vi "scp_send.vi"() -> ()   [LabVIEW 2017]
doc: "Illustrates how to send a file to a remote server via SCP."
uses:
  libssh2/libssh2_session_handshake_tcp.vi
  libssh2/libssh2_init_default.vi
  libssh2/libssh2_session_init_ex.vi
  <vilib>/Utility/tcp.llb/TCP Get Raw Net Object.vi
  libssh2/libssh2_session_handshake_socket.vi
  libssh2/libssh2_userauth_password_ex.vi
  libssh2/libssh2_channel_write_ex.vi
  libssh2/libssh2.lvlib
panel:
  out "size(s)":i32
  in  "data":string="Lorem ipsum dolor sit amet, consetetur sadipscing elitr, sed diam nonumy eirmod tempor invidunt ut labore et dolore magna aliquyam erat, sed diam voluptua. At vero eos et accusam et justo duo dolores et ea rebum. Stet clita kasd gubergren, no sea takimata sanctus est Lorem ipsum dolor sit amet. Lorem ipsum dolor sit amet, consetetur sadipscing elitr, sed diam nonumy eirmod tempor invidunt ut labore et dolore magna aliquyam erat, sed diam voluptua. At vero eos et accusam et justo duo dolores et ea rebum. Stet clita kasd gubergren, no sea takimata sanctus est Lorem ipsum dolor sit amet."
  out "error message":string
  in  "file":string="/"
  out "error out":errorcluster
  in  "password":string
  in  "username":string
  in  "hostname":string
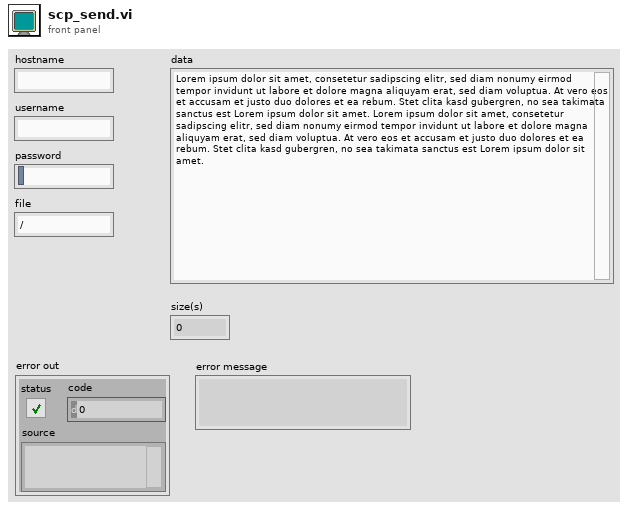
[diagram p1: front panel]
types:
  T1 = typedef "libssh2.lvlib/Session Refnum.ctl" = refnum<k1>
  T2 = typedef "libssh2.lvlib/Channel Refnum.ctl" = refnum<k1>
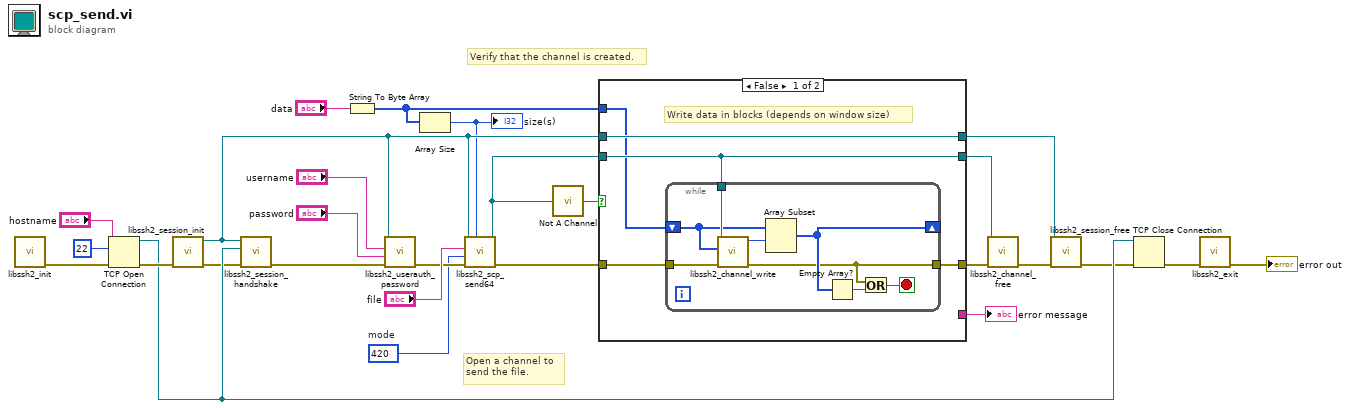
[diagram p0: block diagram]
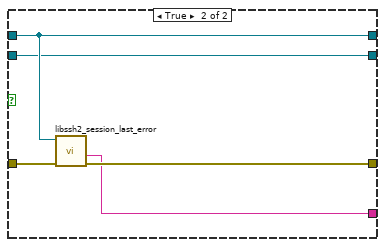
[diagram p2: hidden frame]
diagram:
  w1 = 420  # mode
  # "Verify that the channel is created."
  # "Open a channel to\nsend the file."
  n1 = call-poly "libssh2_init.vi"() -> ("error out"=w26:errorcluster)  [unwired: 11 in]
  n2 = TCP Open Connection(address="hostname", remote port or service name=u16 22, error in (no error)=w26) -> (connection ID=w24:refnum<k5>, error out=w25:errorcluster)  [unwired: 2 in]
  n3 = call "libssh2_session_init.vi"("error in (no error)"=w25) -> ("error out"=w23:errorcluster, "session"=w11:T1)  [unwired: 9 in]
  n4 = call-poly "libssh2_session_handshake.vi"("error in (no error)"=w23, "tcp connection"=w24, "session"=w11) -> ("error out"=w27:errorcluster)  [unwired: 8 in]
  n5 = String To Byte Array(string="data") -> (unsigned byte array=w2:u8[])
  n6 = call "libssh2_userauth_password.vi"("error in (no error)"=w27, "password"="password", "username"="username", "session"=w11) -> ("error out"=w14:errorcluster)  [unwired: 7 in]
  n7 = Array Size(array=w2) -> (size(s)=w4:i32)
  "size(s)" <- w4
  n8 = call "libssh2_scp_send64.vi"("size"=w4, "error in (no error)"=w14, "mode"=w1, "path"="file", "session"=w11) -> ("error out"=w13:errorcluster, "channel"=w8:T2)  [unwired: 5 in]
  n9 = call "Not A Channel.vi"("channel"=w8) -> ("Not a Channel?"=w12:bool)
  n10 = case shown="False" w12 {
    tunnel: w13 -> [w31 w45]
    tunnel: w11 -> [w32 w44]
    tunnel: [w32 w44] -> w10
    tunnel: [w30 w43] -> w5
    tunnel: [_ w42] -> w9
    tunnel: w8 -> [w29 w41]
    tunnel: [w29 w41] -> w7
    tunnel: w2 -> [w28 _]
    frame False {
      # "Write data in blocks (depends on window size)"
      n11 = while {
        tunnel: w31 -> [w40]
        tunnel: [w35] -> w30
        tunnel: w29 -> [w39]
        shift-right: [w37] -> _
        shift-left: w28 -> [w38]
        stop <- w34 stop-if-true
        n12 = call "libssh2_channel_write.vi"("error in (no error)"=w40, "buffer"=w38, "channel"=w39) -> ("error out"=w35:errorcluster, "bytes written"=w33:i32)  [unwired: 7 in]
        n13 = Array Subset(array=w38, index=w33) -> (w37:u8[])  [unwired: 1 in]
        n14 = Empty Array?(array=w37) -> (empty?=w36:bool)
        n15 = Or(x=w35, y=w36) -> (x .or. y?=w34:bool)
      }
    }
    frame True {
      n16 = call "libssh2_session_last_error.vi"("error in (no error)"=w45, "session"=w44) -> ("error out"=w43:errorcluster, "error message"=w42:string)  [unwired: 7 in, 1 out]
    }
  }
  "error message" <- w9
  n17 = call "libssh2_channel_free.vi"("error in (no error)"=w5, "channel"=w7) -> ("error out"=w6:errorcluster)  [unwired: 9 in]
  n18 = call "libssh2_session_free.vi"("error in (no error)"=w6, "session"=w10) -> ("error out"=w17:errorcluster)  [unwired: 9 in]
  n19 = TCP Close Connection(connection ID=w24, error in (no error)=w17) -> (error out=w16:errorcluster)  [unwired: 1 in, 1 out]
  n20 = call "libssh2_exit.vi"("error in (no error)"=w16) -> ("error out"=→"error out":errorcluster)  [unwired: 10 in]
